vi "load_xml.vi"(8 "error in":errorcluster, 10 "child node in":refnum<k20>) -> (0 "error out":errorcluster, 2 "child node out":refnum<k20>, 3 "Counter Settings":T1 {"Array of Counter Settings"."Binwidth (ms)" format="%0.2f"})   [LabVIEW 2012, in "Counter.lvclass"]
doc: "Loads Counter settings from xml in the format:\n\n<Enable>%b</Enable>\n<ArrayOfCounterSettings>\n<counter>\n<CounterChannel>%s</CounterChannel>\n<TimeBinClockChannel>%s</TimeBinClockChannel>\n<binWidth units=\"ms\">%f</binWidth>\n</counter>\n</ArrayOfCounterSettings>\n\nMTL 2013 Jan 1"
uses:
  Counter.lvclass
  Counter_Settings_Control.ctl
  <vilib>/xml/Close Reference(Node).vi
  <resource>/objmgr/DOMUserDefRef.rc
  <vilib>/xml/NI_XML.lvlib
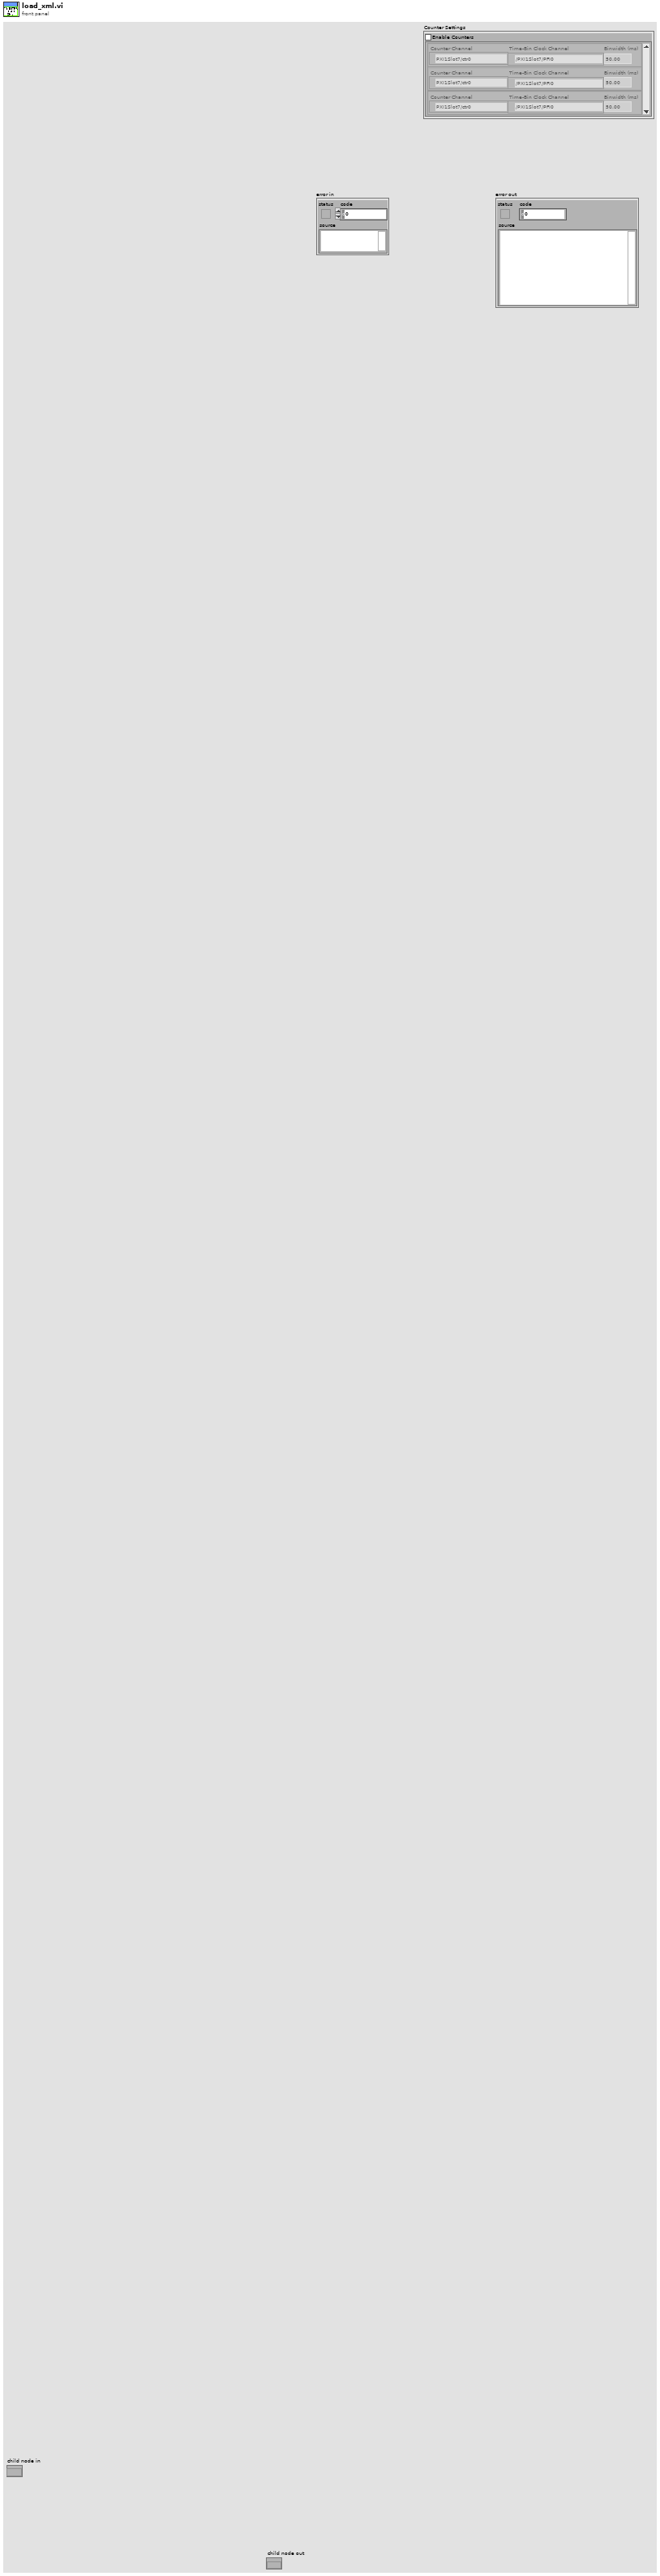
[diagram p1: front panel]
types:
  T1 = typedef "Counter.lvclass/Counter_Settings_Control.ctl" = cluster{"Enable Counters":bool, "Array of Counter Settings":cluster{"Counter Channel":tag, "Time-Bin Clock Channel":tag, "Binwidth (ms)":dbl}[]}
  T2 = cluster{"Counter Channel":tag, "Time-Bin Clock Channel":tag, "Binwidth (ms)":dbl}
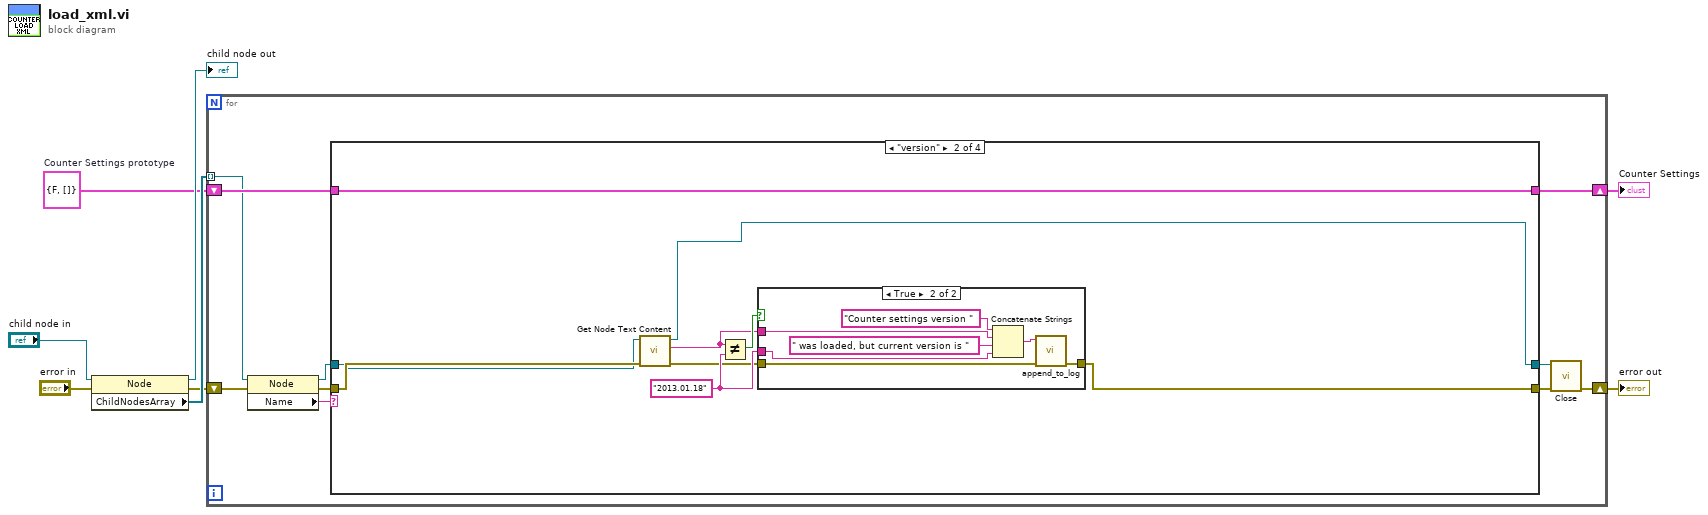
[diagram p0: block diagram]
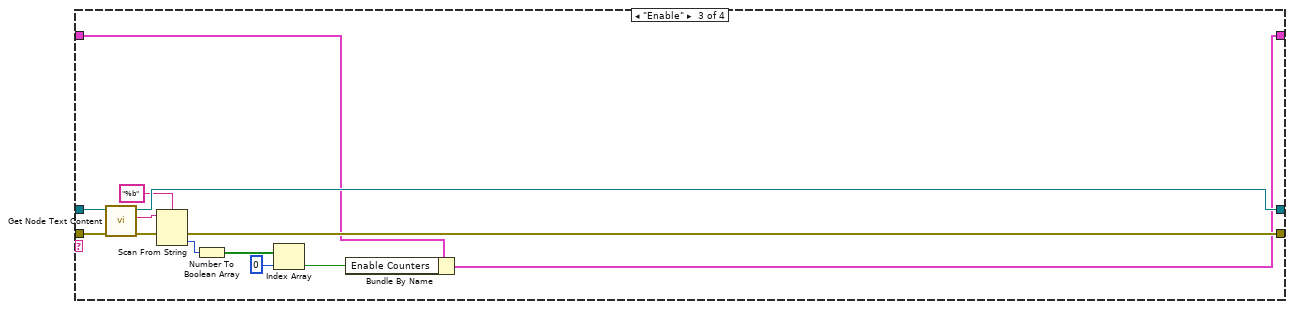
[diagram p4: hidden frame]
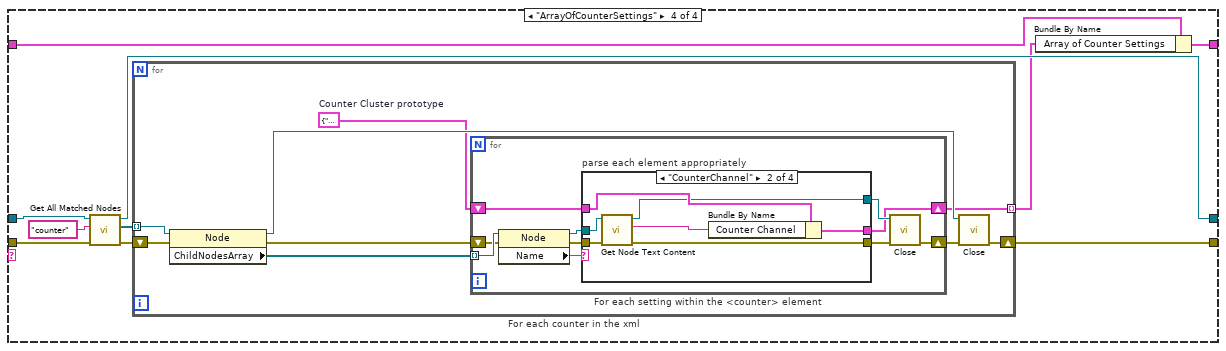
[diagram p5: hidden frame]
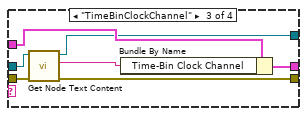
[diagram p7: hidden frame]
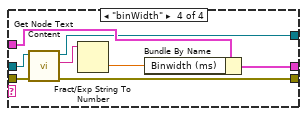
[diagram p8: hidden frame]
diagram:
  w1 = T1 {"Enable Counters"=FALSE, "Array of Counter Settings"=[]}  # Counter Settings prototype
  n1 = property class="Node"(reference="child node in", error in="error in") -> (reference out=→"child node out":refnum<k20>, error out=w6:errorcluster, "ChildNodesArray"=w8:refnum<k20>[])
  n2 = for {
    tunnel: w8 -> [w9] mode=indexing
    shift-right: [w15] -> w2
    shift-left: w1 -> [w16]
    shift-right: [w12] -> w3
    shift-left: w6 -> [w10]
    n3 = property class="Node"(reference=w9, error in=w10) -> (reference out=w17:refnum<k20>, error out=w13:errorcluster, "Name"=w18:string)
    n4 = case shown="\"version\"" w18 {
      tunnel: w17 -> [w20 w24 w50 w58]
      tunnel: w16 -> [w21 w26 w40 w61]
      tunnel: [w21 w26 w39 w60] -> w15
      tunnel: [w20 w23 w51 w57] -> w14
      tunnel: w13 -> [w19 w25 w49 w56]
      tunnel: [w19 w22 w41 w53] -> w11
      frame "None", Default {
      }
      frame "version" {
        w28 = "2013.01.18" ("y")
        n5 = call <vilib>:"Get Node Text Content.vi"("error in (no error)"=w25, "node in"=w24) -> ("error out"=w27:errorcluster, "node text"=w29:string, "node out"=w23:refnum<k20>)  [unwired: 7 in]
        n6 = Not Equal?(x=w29, y=w28) -> (x != y?=w30:bool)
        n7 = case shown="True" w30 {
          tunnel: w29 -> [_ w37]
          tunnel: w28 -> [_ w35]
          tunnel: w27 -> [w31 w33]
          tunnel: [w31 w32] -> w22
          frame False {
          }
          frame True {
            n8 = Concatenate Strings("Counter settings version " ("string"), w37, " was loaded, but current version is " ("string"), w35) -> (w34:string)
            n9 = call "append_to_log.vi"("error in"=w33, "string"=w34) -> ("error out"=w32:errorcluster)  [unwired: 8 in, 1 out]
          }
        }
      }
      frame "Enable" {
        n10 = call <vilib>:"Get Node Text Content.vi"("error in (no error)"=w49, "node in"=w50) -> ("error out"=w42:errorcluster, "node text"=w43:string, "node out"=w51:refnum<k20>)  [unwired: 7 in]
        n11 = Scan From String(format string="%b", input string=w43, error in=w42) -> (error out=w41:errorcluster, output 1=w44:i32)  [unwired: 2 in, 2 out]
        n12 = Number To Boolean Array(number=w44) -> (Boolean array=w48:bool[])
        n13 = Index Array(array=w48, index=0) -> (element=w46:bool)
        n14 = Bundle By Name(cluster=w40, "Enable Counters"=w46) -> (w39:T1)
      }
      frame "ArrayOfCounterSettings" {
        n15 = call <vilib>:"Get All Matched Nodes.vi"("error in (no error)"=w56, "XPath expression"="counter", "node in"=w58) -> ("error out"=w54:errorcluster, "node result array"=w59:refnum<k20>[], "node out"=w57:refnum<k20>)  [unwired: 6 in]
        n16 = for "For each counter in the xml" {
          tunnel: w59 -> [w69] mode=indexing
          shift-right: [w70] -> w53
          shift-left: w54 -> [w67]
          tunnel: [w62] -> w52 mode=indexing
          w63 = T2 {"Counter Channel"="", "Time-Bin Clock Channel"="", "Binwidth (ms)"=0.0}  # Counter Cluster prototype
          n17 = property class="Node"(reference=w69, error in=w67) -> (reference out=w65:refnum<k20>, error out=w66:errorcluster, "ChildNodesArray"=w68:refnum<k20>[])
          n18 = for "For each setting within the <counter> element" {
            tunnel: w68 -> [w80] mode=indexing
            shift-right: [w75] -> w64
            shift-left: w66 -> [w78]
            shift-right: [w71] -> w62
            shift-left: w63 -> [w73]
            n19 = property class="Node"(reference=w80, error in=w78) -> (reference out=w74:refnum<k20>, error out=w77:errorcluster, "Name"=w79:string)
            n20 = case "parse each element appropriately" shown="\"CounterChannel\"" w79 {
              tunnel: w77 -> [w83 w89 w96 w104]
              tunnel: [w83 w86 w93 w102] -> w76
              tunnel: w74 -> [w82 w90 w97 w105]
              tunnel: w73 -> [w81 w88 w95 w103]
              tunnel: [w82 w85 w92 w101] -> w72
              tunnel: [w81 w84 w91 w98] -> w71
              frame "None", Default {
              }
              frame "CounterChannel" {
                n21 = call <vilib>:"Get Node Text Content.vi"("error in (no error)"=w89, "node in"=w90) -> ("error out"=w86:errorcluster, "node text"=w87:string, "node out"=w85:refnum<k20>)  [unwired: 7 in]
                n22 = Bundle By Name(cluster=w88, "Counter Channel"=w87) -> (w84:T2)
              }
              frame "TimeBinClockChannel" {
                n23 = call <vilib>:"Get Node Text Content.vi"("error in (no error)"=w96, "node in"=w97) -> ("error out"=w93:errorcluster, "node text"=w94:string, "node out"=w92:refnum<k20>)  [unwired: 7 in]
                n24 = Bundle By Name(cluster=w95, "Time-Bin Clock Channel"=w94) -> (w91:T2)
              }
              frame "binWidth" {
                n25 = call <vilib>:"Get Node Text Content.vi"("error in (no error)"=w104, "node in"=w105) -> ("error out"=w102:errorcluster, "node text"=w100:string, "node out"=w101:refnum<k20>)  [unwired: 7 in]
                n26 = Fract/Exp String To Number(string=w100) -> (number=w99:dbl)  [unwired: 3 in, 1 out]
                n27 = Bundle By Name(cluster=w103, "Binwidth (ms)"=w99) -> (w98:T2)
              }
            }
            n28 = call-poly <vilib>:"Close.vi"("error in (no error)"=w76, "node"=w72) -> ("error out"=w75:errorcluster)  [unwired: 7 in]
          }
          n29 = call-poly <vilib>:"Close.vi"("error in (no error)"=w64, "node"=w65) -> ("error out"=w70:errorcluster)  [unwired: 7 in]
        }
        n30 = Bundle By Name(cluster=w61, "Array of Counter Settings"=w52) -> (w60:T1)
      }
    }
    n31 = call-poly <vilib>:"Close.vi"("error in (no error)"=w11, "node"=w14) -> ("error out"=w12:errorcluster)  [unwired: 7 in]
  }
  "error out" <- w3
  "Counter Settings" <- w2
